vi "Ex4_WhileLoop.vi"() -> ()   [LabVIEW 2024]
panel:
  out "Numeric":i32
  in  "stop":bool
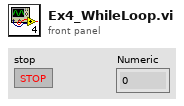
[diagram p1: front panel]
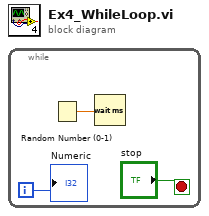
[diagram p0: block diagram]
diagram:
  n1 = while {
    i -> [w2]
    stop <- "stop" stop-if-true
    n2 = Random Number (0-1)() -> (number: 0 to 1=w1:dbl)
    n3 = Wait (ms)(milliseconds to wait=w1) -> ()  [unwired: 1 out]
    "Numeric" <- w2
  }
